vi "ProyectoAndres.vi"() -> ()   [LabVIEW 2013]
uses:
  <vilib>/Instr/_visa.llb/VISA Configure Serial Port (Instr).vi
panel:
  in  "sample waiting time":dbl(knob) scale=0.0..500.0
  out "Corte":bool
  out "Corte":string
  out "RPM":i32(graph)
  out "Temperatura":i32(graph)
  out "Nivel":i32(graph)
  out "NIVEL":dbl(slide) scale=0.0..30.0
  out "RPM":dbl(knob) scale=0.0..100.0
  out "Temperatura":dbl(slide) scale=0.0..300.0
  out "RPM":string
  out "TEMPERATURA":string
  out "ERROR":string
  out "OUTPUT":string
  out "ALTURA":string
  in  "INPUT":refnum<visa-resource-name>
  in  "stop":bool
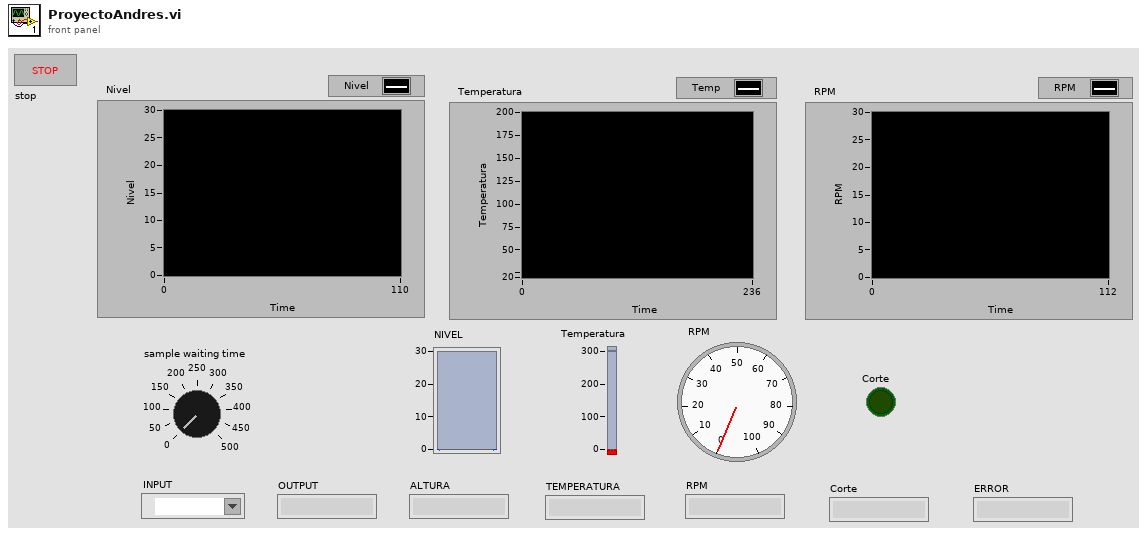
[diagram p1: front panel]
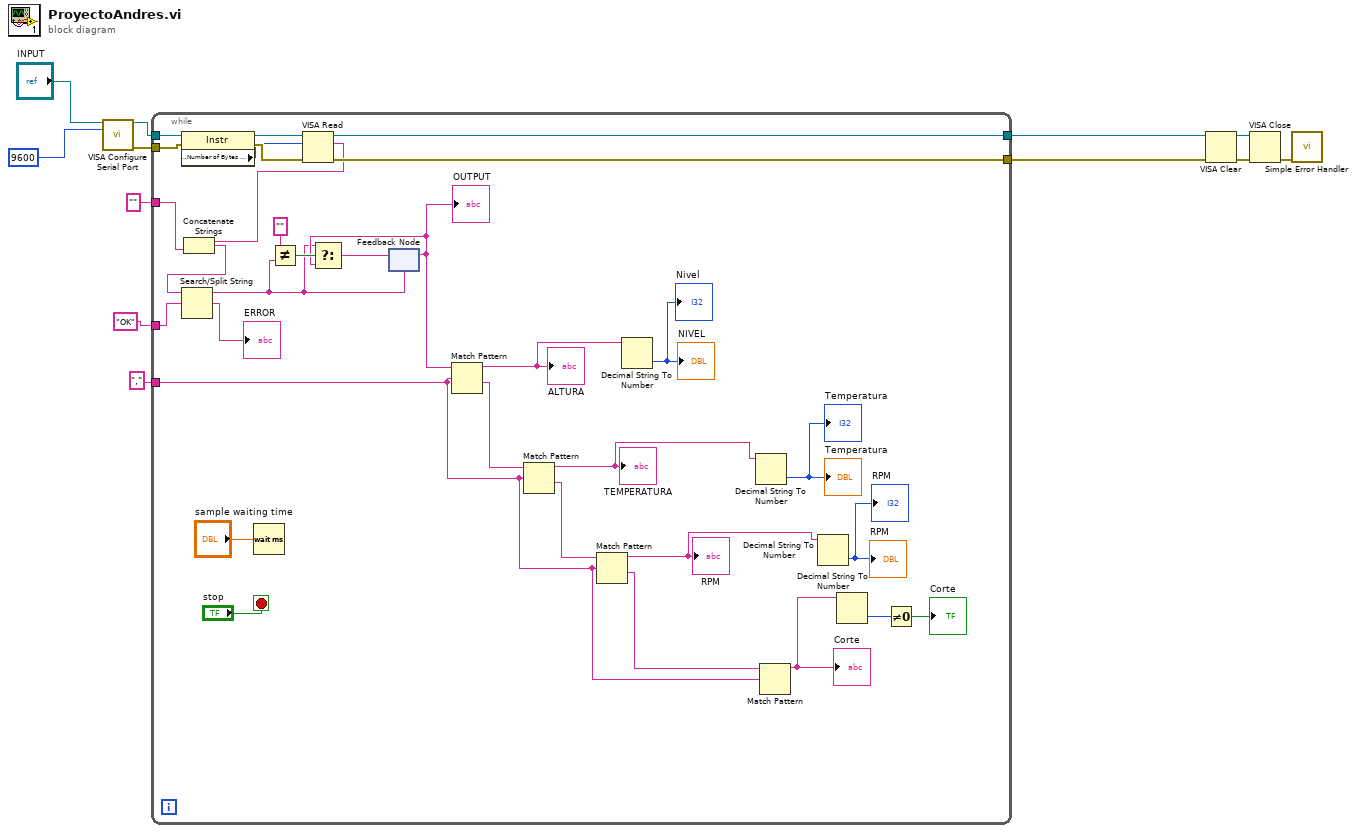
[diagram p0: block diagram]
diagram:
  n1 = call-poly "VISA Configure Serial Port"("VISA resource name"="INPUT", "baud rate (9600)"=u32 9600) -> ("VISA resource name out"=w11:refnum<visa-resource-name>, "error out"=w10:errorcluster)  [unwired: 12 in]
  n2 = while {
    tunnel: w11 -> [w43]
    tunnel: w10 -> [w42]
    tunnel: [w38] -> w4
    tunnel: [w37] -> w3
    tunnel: "" ("string") -> [w36]
    tunnel: "OK" ("search string/char (-)") -> [w33]
    tunnel: "," ("regular expression") -> [w22]
    stop <- "stop" stop-if-true
    n3 = property class="Instr"(reference=w43, error in=w42) -> (reference out=w41:refnum<visa-resource-name>, error out=w40:errorcluster, "Serial Settings:Number of Bytes at Serial Port"=w39:u32)
    n4 = Wait (ms)(milliseconds to wait="sample waiting time") -> ()  [unwired: 1 out]
    n5 = VISA Read(VISA resource name=w41, byte count=w39, error in (no error)=w40) -> (VISA resource name out=w38:refnum<visa-resource-name>, read buffer=w35:string, error out=w37:errorcluster)  [unwired: 1 out]
    n6 = Concatenate Strings(w35, w36) -> (w34:string)
    n7 = Search/Split String(string=w34, search string/char (-)=w33) -> (substring before match=w13:string, match + rest of string=→"ERROR":string)  [unwired: 1 in, 1 out]
    n8 = Not Equal?(x="" ("y"), y=w13) -> (x != y?=w16:bool)
    n9 = feedback #1(w13) -> (w15:string)
    "OUTPUT" <- w15
    n10 = Select(t=w13, s=w16, f=w15) -> (s? t:f=w17:string)
    n11 = feedback-in #1(w17) -> ()
    n12 = Match Pattern(string=w15, regular expression=w22) -> (before substring=w29:string, after substring=w31:string)  [unwired: 1 in, 2 out]
    "ALTURA" <- w29
    n13 = Match Pattern(string=w31, regular expression=w22) -> (before substring=w28:string, after substring=w30:string)  [unwired: 1 in, 2 out]
    "TEMPERATURA" <- w28
    n14 = Match Pattern(string=w30, regular expression=w22) -> (before substring=w27:string, after substring=w23:string)  [unwired: 1 in, 2 out]
    "RPM" <- w27
    n15 = Decimal String To Number(string=w29) -> (number=→"NIVEL" →"Nivel":i32)  [unwired: 2 in, 1 out]
    n16 = Decimal String To Number(string=w28) -> (number=→"Temperatura" →"Temperatura":i32)  [unwired: 2 in, 1 out]
    n17 = Match Pattern(string=w23, regular expression=w22) -> (before substring=w21:string)  [unwired: 1 in, 3 out]
    "Corte" <- w21
    n18 = Decimal String To Number(string=w27) -> (number=→"RPM" →"RPM":i32)  [unwired: 2 in, 1 out]
    n19 = Decimal String To Number(string=w21) -> (number=w19:i32)  [unwired: 2 in, 1 out]
    n20 = Not Equal To 0?(x=w19) -> (x != 0?=→"Corte":bool)
  }
  n21 = VISA Clear(VISA resource name=w4, error in (no error)=w3) -> (VISA resource name out=w2:refnum<visa-resource-name>, error out=w1:errorcluster)
  n22 = VISA Close(VISA resource name=w2, error in (no error)=w1) -> (error out=w9:errorcluster)
  n23 = call <vilib>:"Simple Error Handler.vi"("error in (no error)"=w9) -> ()  [unwired: 4 in, 5 out]
